vi "Load AI Driver.vi"(8 "error in (no error)":errorcluster, 9 "Config Path":path, 10 "Section":string, 11 "SIm AI Factory in":refnum<class "SIm AI Factory.lvclass">) -> (0 "error out":errorcluster, 2 "AI Driver.lvclass":refnum<class "AI Driver.lvclass">)   [LabVIEW 2022 SP3, in "SIm AI Factory.lvclass"]
uses:
  SIm AI Factory.lvclass
  SIm AI Factory.lvclass/SIm AI Factory.ctl
  SIM AI Driver/SIM AI Driver.lvclass
  C:/XY Stage/IO Monitor/SIM AI Driver/SIM AI Driver.lvclass
  C:/XY Stage/IO Monitor/AI Driver/AI Driver.lvclass
  AI Driver/AI Driver.lvclass
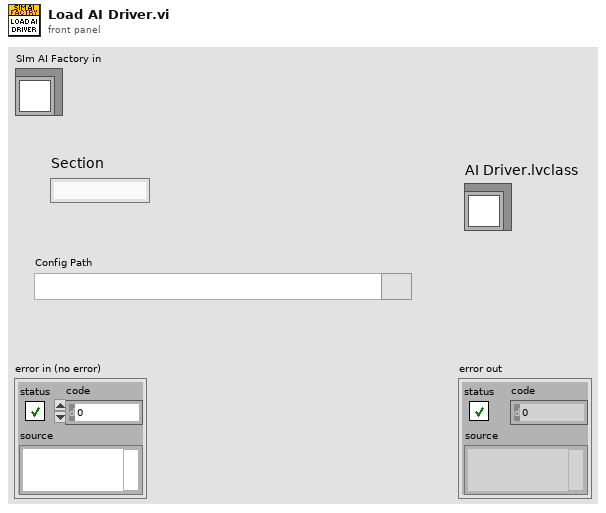
[diagram p1: front panel]
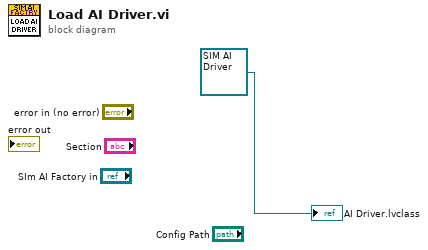
[diagram p0: block diagram]
diagram:
  "AI Driver.lvclass" <- refnum<class "SIM AI Driver.lvclass"> refnum ("SIM AI Driver.lvclass")
